vi "RubikTurnFSM(vgl. RubikMove).vi"(1 "Turn":T1) -> ()   [LabVIEW 2017]
uses:
  Controls/RubikMoves.ctl
  Projekt-RubikLibrary/ServoEnumControl.ctl
  Projekt-RubikLibrary/ServoAbsAngleControl.ctl
  8eb4d94e-5852-4223-b3f1-68aace851966.vi
  Projekt-RubikLibrary/RubikLibrary.lvlib
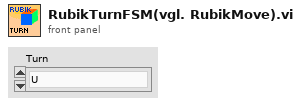
[diagram p1: front panel]
types:
  T1 = typedef "RubikMoves.ctl" = enum16{"U", "U'", "F", "F'", "D", "D'", "B", "B'", "L", "L'", "R", "R'"}
  T2 = typedef "RubikLibrary.lvlib/ServoEnumControl.ctl" = enum16{"Left Servo", "Front Servo", "Right Servo"}
  T3 = typedef "RubikLibrary.lvlib/ServoAbsAngleControl.ctl" = enum16{"-90°", "0°", "+90°"}
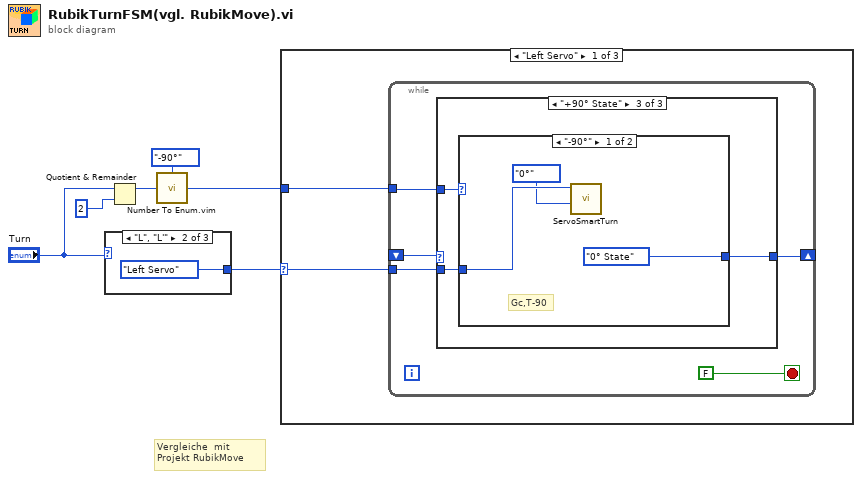
[diagram p0: block diagram]
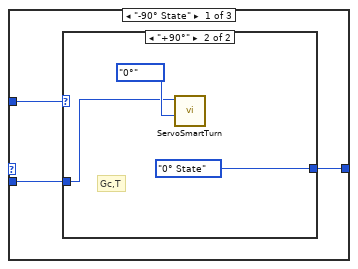
[diagram p2: hidden frame]
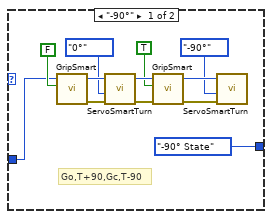
[diagram p3: hidden frame]
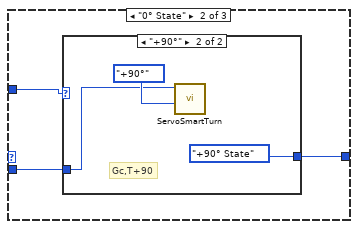
[diagram p4: hidden frame]
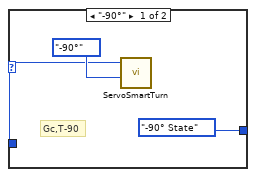
[diagram p5: hidden frame]
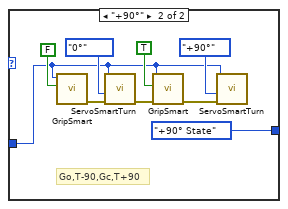
[diagram p6: hidden frame]
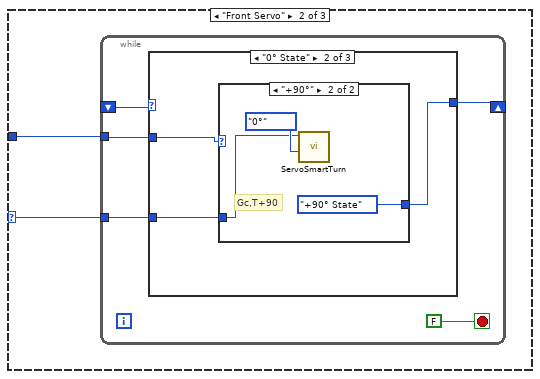
[diagram p7: hidden frame]
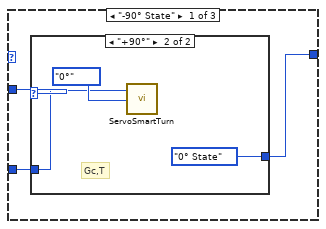
[diagram p8: hidden frame]
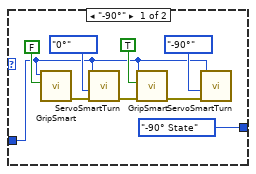
[diagram p9: hidden frame]
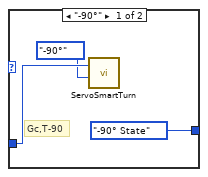
[diagram p10: hidden frame]
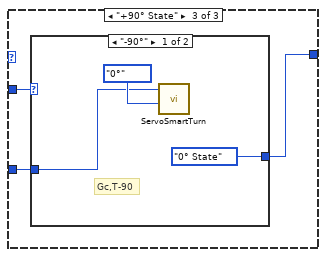
[diagram p11: hidden frame]
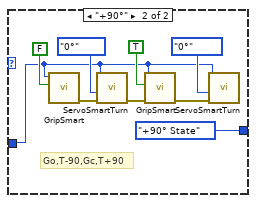
[diagram p12: hidden frame]
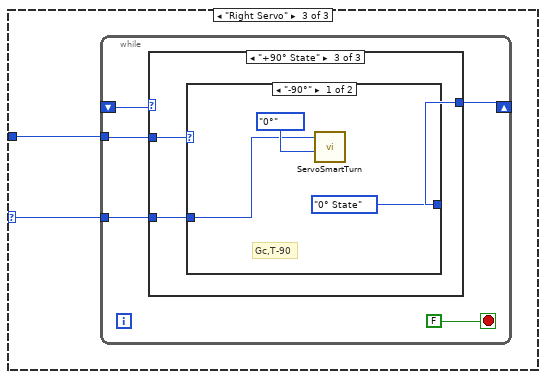
[diagram p13: hidden frame]
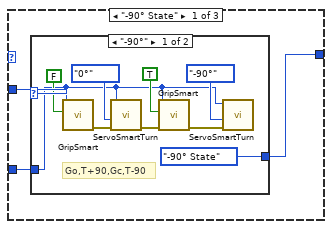
[diagram p14: hidden frame]
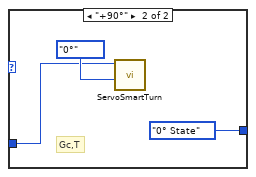
[diagram p15: hidden frame]
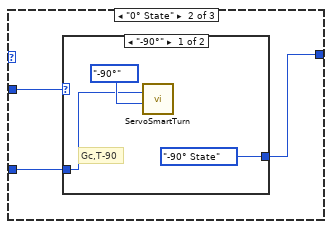
[diagram p16: hidden frame]
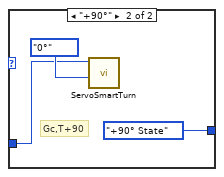
[diagram p17: hidden frame]
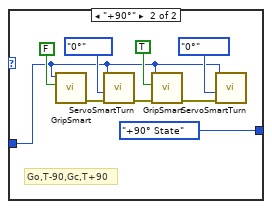
[diagram p18: hidden frame]
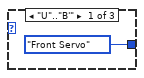
[diagram p19: hidden frame]
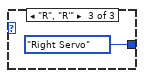
[diagram p20: hidden frame]
diagram:
  # "Vergleiche  mit Projekt RubikMove"
  n1 = case shown="\"L\", \"L'\"" "Turn" {
    tunnel: [ServoEnumControl."Front Servo" ("Servo Enum") ServoEnumControl."Left Servo" ("Servo Enum") ServoEnumControl."Right Servo" ("Servo Enum")] -> w6
    frame "U".."B'" {
    }
    frame "L", "L'" {
    }
    frame "R", "R'" {
    }
  }
  n2 = Quotient & Remainder(x="Turn", y=2) -> (x-y*floor(x/y)=w3:i32)  [unwired: 1 out]
  n3 = call "Number To Enum.vim"("number"=w3, "enum type"=enum16{"-90°", "+90°"}."-90°" ("Turn by")) -> ("number as enum"=w1:enum16{"-90°", "+90°"})
  n4 = case shown="\"Left Servo\"" w6 {
    selector: w6 -> [w10 w56 w102]
    tunnel: w1 -> [w11 w57 w103]
    frame "Left Servo" {
      n5 = while {
        shift-right: [w15] -> _
        shift-left: _ -> [w16]
        tunnel: w11 -> [w13]
        tunnel: w10 -> [w12]
        stop <- FALSE stop-if-true
        n6 = case shown="\"+90° State\"" w16 {
          tunnel: [w19 w34 w43] -> w15
          tunnel: w13 -> [w18 w33 w42]
          tunnel: w12 -> [w17 w32 w41]
          frame "-90° State" {
            n7 = case shown="\"+90°\"" w18 {
              tunnel: [enum16{"-90° State", "0° State", "+90° State"}."-90° State" ("Enum 2") enum16{"-90° State", "0° State", "+90° State"}."0° State" ("Enum 2")] -> w19
              tunnel: w17 -> [w23 w29]
              frame "-90°" {
                # "Go,T+90,Gc,T-90"
                n8 = call "GripSmart.vi"("Turn to (in)"=FALSE, "Servo"=w23) -> ("error out"=w26:errorcluster)  [unwired: 8 in, 1 out]
                n9 = call "ServoSmartTurn.vi"("error in"=w26, "Turn to (in)"=ServoAbsAngleControl."0°" ("Turn to"), "Servo"=w23) -> ("error out"=w25:errorcluster)  [unwired: 7 in, 1 out]
                n10 = call "GripSmart.vi"("error in"=w25, "Turn to (in)"=TRUE, "Servo"=w23) -> ("error out"=w24:errorcluster)  [unwired: 7 in, 1 out]
                n11 = call "ServoSmartTurn.vi"("error in"=w24, "Turn to (in)"=ServoAbsAngleControl."-90°" ("Turn to"), "Servo"=w23) -> ()  [unwired: 7 in, 2 out]
              }
              frame "+90°" {
                # "Gc,T"
                n12 = call "ServoSmartTurn.vi"("Turn to (in)"=ServoAbsAngleControl."0°" ("Turn to"), "Servo"=w29) -> ()  [unwired: 8 in, 2 out]
              }
            }
          }
          frame "0° State" {
            n13 = case shown="\"+90°\"" w33 {
              tunnel: [enum16{"-90° State", "0° State", "+90° State"}."-90° State" ("Enum 2") enum16{"-90° State", "0° State", "+90° State"}."+90° State" ("Enum 2")] -> w34
              tunnel: w32 -> [w35 w38]
              frame "-90°" {
                # "Gc,T-90"
                n14 = call "ServoSmartTurn.vi"("Turn to (in)"=ServoAbsAngleControl."-90°" ("Turn to"), "Servo"=w35) -> ()  [unwired: 8 in, 2 out]
              }
              frame "+90°" {
                # "Gc,T+90"
                n15 = call "ServoSmartTurn.vi"("Turn to (in)"=ServoAbsAngleControl."+90°" ("Turn to"), "Servo"=w38) -> ()  [unwired: 8 in, 2 out]
              }
            }
          }
          frame "+90° State" {
            n16 = case shown="\"-90°\"" w42 {
              tunnel: [enum16{"-90° State", "0° State", "+90° State"}."0° State" ("Enum 2") enum16{"-90° State", "0° State", "+90° State"}."+90° State" ("Enum 2")] -> w43
              tunnel: w41 -> [w45 w47]
              frame "-90°" {
                # "Gc,T-90"
                n17 = call "ServoSmartTurn.vi"("Turn to (in)"=ServoAbsAngleControl."0°" ("Turn to"), "Servo"=w45) -> ()  [unwired: 8 in, 2 out]
              }
              frame "+90°" {
                # "Go,T-90,Gc,T+90"
                n18 = call "GripSmart.vi"("Turn to (in)"=FALSE, "Servo"=w47) -> ("error out"=w53:errorcluster)  [unwired: 8 in, 1 out]
                n19 = call "ServoSmartTurn.vi"("error in"=w53, "Turn to (in)"=ServoAbsAngleControl."0°" ("Turn to"), "Servo"=w47) -> ("error out"=w52:errorcluster)  [unwired: 7 in, 1 out]
                n20 = call "GripSmart.vi"("error in"=w52, "Turn to (in)"=TRUE, "Servo"=w47) -> ("error out"=w51:errorcluster)  [unwired: 7 in, 1 out]
                n21 = call "ServoSmartTurn.vi"("error in"=w51, "Turn to (in)"=ServoAbsAngleControl."+90°" ("Turn to"), "Servo"=w47) -> ()  [unwired: 7 in, 2 out]
              }
            }
          }
        }
      }
    }
    frame "Front Servo" {
      n22 = while {
        shift-right: [w61] -> _
        shift-left: _ -> [w62]
        tunnel: w57 -> [w59]
        tunnel: w56 -> [w58]
        stop <- FALSE stop-if-true
        n23 = case shown="\"0° State\"" w62 {
          tunnel: [w65 w80 w89] -> w61
          tunnel: w59 -> [w64 w79 w88]
          tunnel: w58 -> [w63 w78 w87]
          frame "-90° State" {
            n24 = case shown="\"+90°\"" w64 {
              tunnel: [enum16{"-90° State", "0° State", "+90° State"}."-90° State" ("Enum 2") enum16{"-90° State", "0° State", "+90° State"}."0° State" ("Enum 2")] -> w65
              tunnel: w63 -> [w66 w75]
              frame "-90°" {
                n25 = call "GripSmart.vi"("Turn to (in)"=FALSE, "Servo"=w66) -> ("error out"=w72:errorcluster)  [unwired: 8 in, 1 out]
                n26 = call "ServoSmartTurn.vi"("error in"=w72, "Turn to (in)"=ServoAbsAngleControl."0°" ("Turn to"), "Servo"=w66) -> ("error out"=w71:errorcluster)  [unwired: 7 in, 1 out]
                n27 = call "GripSmart.vi"("error in"=w71, "Turn to (in)"=TRUE, "Servo"=w66) -> ("error out"=w70:errorcluster)  [unwired: 7 in, 1 out]
                n28 = call "ServoSmartTurn.vi"("error in"=w70, "Turn to (in)"=ServoAbsAngleControl."-90°" ("Turn to"), "Servo"=w66) -> ()  [unwired: 7 in, 2 out]
              }
              frame "+90°" {
                # "Gc,T"
                n29 = call "ServoSmartTurn.vi"("Turn to (in)"=ServoAbsAngleControl."0°" ("Turn to"), "Servo"=w75) -> ()  [unwired: 8 in, 2 out]
              }
            }
          }
          frame "0° State" {
            n30 = case shown="\"+90°\"" w79 {
              tunnel: [enum16{"-90° State", "0° State", "+90° State"}."-90° State" ("Enum 2") enum16{"-90° State", "0° State", "+90° State"}."+90° State" ("Enum 2")] -> w80
              tunnel: w78 -> [w82 w84]
              frame "-90°" {
                # "Gc,T-90"
                n31 = call "ServoSmartTurn.vi"("Turn to (in)"=ServoAbsAngleControl."-90°" ("Turn to"), "Servo"=w82) -> ()  [unwired: 8 in, 2 out]
              }
              frame "+90°" {
                # "Gc,T+90"
                n32 = call "ServoSmartTurn.vi"("Turn to (in)"=ServoAbsAngleControl."0°" ("Turn to"), "Servo"=w84) -> ()  [unwired: 8 in, 2 out]
              }
            }
          }
          frame "+90° State" {
            n33 = case shown="\"-90°\"" w88 {
              tunnel: [enum16{"-90° State", "0° State", "+90° State"}."0° State" ("Enum 2") enum16{"-90° State", "0° State", "+90° State"}."+90° State" ("Enum 2")] -> w89
              tunnel: w87 -> [w90 w93]
              frame "-90°" {
                # "Gc,T-90"
                n34 = call "ServoSmartTurn.vi"("Turn to (in)"=ServoAbsAngleControl."0°" ("Turn to"), "Servo"=w90) -> ()  [unwired: 8 in, 2 out]
              }
              frame "+90°" {
                # "Go,T-90,Gc,T+90"
                n35 = call "GripSmart.vi"("Turn to (in)"=FALSE, "Servo"=w93) -> ("error out"=w99:errorcluster)  [unwired: 8 in, 1 out]
                n36 = call "ServoSmartTurn.vi"("error in"=w99, "Turn to (in)"=ServoAbsAngleControl."0°" ("Turn to"), "Servo"=w93) -> ("error out"=w98:errorcluster)  [unwired: 7 in, 1 out]
                n37 = call "GripSmart.vi"("error in"=w98, "Turn to (in)"=TRUE, "Servo"=w93) -> ("error out"=w97:errorcluster)  [unwired: 7 in, 1 out]
                n38 = call "ServoSmartTurn.vi"("error in"=w97, "Turn to (in)"=ServoAbsAngleControl."0°" ("Turn to"), "Servo"=w93) -> ()  [unwired: 7 in, 2 out]
              }
            }
          }
        }
      }
    }
    frame "Right Servo" {
      n39 = while {
        shift-right: [w107] -> _
        shift-left: _ -> [w108]
        tunnel: w103 -> [w105]
        tunnel: w102 -> [w104]
        stop <- FALSE stop-if-true
        n40 = case shown="\"+90° State\"" w108 {
          tunnel: [w111 w126 w135] -> w107
          tunnel: w105 -> [w110 w125 w134]
          tunnel: w104 -> [w109 w124 w133]
          frame "-90° State" {
            n41 = case shown="\"-90°\"" w110 {
              tunnel: [enum16{"-90° State", "0° State", "+90° State"}."-90° State" ("Enum 2") enum16{"-90° State", "0° State", "+90° State"}."0° State" ("Enum 2")] -> w111
              tunnel: w109 -> [w112 w121]
              frame "-90°" {
                # "Go,T+90,Gc,T-90"
                n42 = call "GripSmart.vi"("Turn to (in)"=FALSE, "Servo"=w112) -> ("error out"=w118:errorcluster)  [unwired: 8 in, 1 out]
                n43 = call "ServoSmartTurn.vi"("error in"=w118, "Turn to (in)"=ServoAbsAngleControl."0°" ("Turn to"), "Servo"=w112) -> ("error out"=w117:errorcluster)  [unwired: 7 in, 1 out]
                n44 = call "GripSmart.vi"("error in"=w117, "Turn to (in)"=TRUE, "Servo"=w112) -> ("error out"=w116:errorcluster)  [unwired: 7 in, 1 out]
                n45 = call "ServoSmartTurn.vi"("error in"=w116, "Turn to (in)"=ServoAbsAngleControl."-90°" ("Turn to"), "Servo"=w112) -> ()  [unwired: 7 in, 2 out]
              }
              frame "+90°" {
                # "Gc,T"
                n46 = call "ServoSmartTurn.vi"("Turn to (in)"=ServoAbsAngleControl."0°" ("Turn to"), "Servo"=w121) -> ()  [unwired: 8 in, 2 out]
              }
            }
          }
          frame "0° State" {
            n47 = case shown="\"-90°\"" w125 {
              tunnel: [enum16{"-90° State", "0° State", "+90° State"}."-90° State" ("Enum 2") enum16{"-90° State", "0° State", "+90° State"}."+90° State" ("Enum 2")] -> w126
              tunnel: w124 -> [w127 w130]
              frame "-90°" {
                # "Gc,T-90"
                n48 = call "ServoSmartTurn.vi"("Turn to (in)"=ServoAbsAngleControl."-90°" ("Turn to"), "Servo"=w127) -> ()  [unwired: 8 in, 2 out]
              }
              frame "+90°" {
                # "Gc,T+90"
                n49 = call "ServoSmartTurn.vi"("Turn to (in)"=ServoAbsAngleControl."0°" ("Turn to"), "Servo"=w130) -> ()  [unwired: 8 in, 2 out]
              }
            }
          }
          frame "+90° State" {
            n50 = case shown="\"-90°\"" w134 {
              tunnel: [enum16{"-90° State", "0° State", "+90° State"}."0° State" ("Enum 2") enum16{"-90° State", "0° State", "+90° State"}."+90° State" ("Enum 2")] -> w135
              tunnel: w133 -> [w136 w139]
              frame "-90°" {
                # "Gc,T-90"
                n51 = call "ServoSmartTurn.vi"("Turn to (in)"=ServoAbsAngleControl."0°" ("Turn to"), "Servo"=w136) -> ()  [unwired: 8 in, 2 out]
              }
              frame "+90°" {
                # "Go,T-90,Gc,T+90"
                n52 = call "GripSmart.vi"("Turn to (in)"=FALSE, "Servo"=w139) -> ("error out"=w145:errorcluster)  [unwired: 8 in, 1 out]
                n53 = call "ServoSmartTurn.vi"("error in"=w145, "Turn to (in)"=ServoAbsAngleControl."0°" ("Turn to"), "Servo"=w139) -> ("error out"=w144:errorcluster)  [unwired: 7 in, 1 out]
                n54 = call "GripSmart.vi"("error in"=w144, "Turn to (in)"=TRUE, "Servo"=w139) -> ("error out"=w143:errorcluster)  [unwired: 7 in, 1 out]
                n55 = call "ServoSmartTurn.vi"("error in"=w143, "Turn to (in)"=ServoAbsAngleControl."0°" ("Turn to"), "Servo"=w139) -> ()  [unwired: 7 in, 2 out]
              }
            }
          }
        }
      }
    }
  }
